vi "SSL_CTX_free.vi"(8 "error in (no error)":errorcluster, 11 "SSL-Context in":refnum<class "SSL-Context.lvclass">) -> (0 "error out":errorcluster)   [LabVIEW 2013, in "SSL_Lib.lvlib" / "SSL-Context.lvclass"]
uses:
  SSL-Context.lvclass
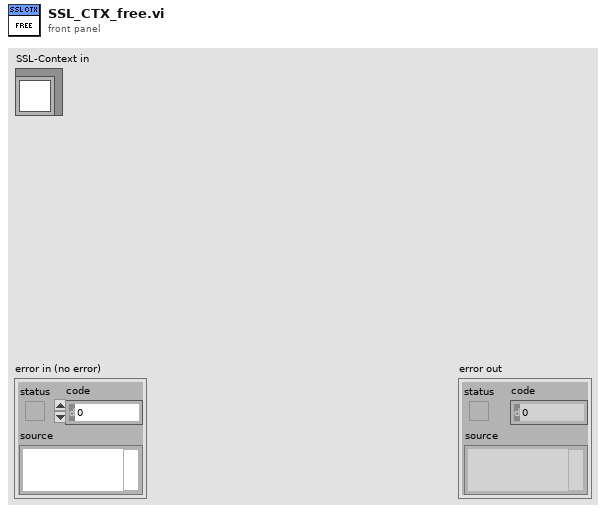
[diagram p1: front panel]
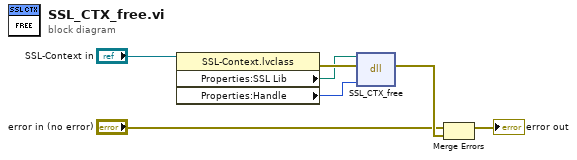
[diagram p0: block diagram]
diagram:
  n1 = property class="SSL-Context.lvclass"(reference="SSL-Context in") -> (error out=w6:errorcluster, "Properties:SSL Lib"=w5:path, "Properties:Handle"=w4:u64)  [unwired: 1 in, 1 out]
  n2 = dll-call lib="C:/Program Files (x86)/National Instruments/Shared/nissl/NIssleay32.dll" fn="SSL_CTX_free"(path in=w5, error in=w6, "*SSL CTX"=w4) -> (error out=w3:errorcluster)  [unwired: 3 in, 1 out]
  n3 = Merge Errors("error in (no error)", w3) -> (→"error out":errorcluster)
